vi "TDMS Write Through Publisher test.vi"() -> ()   [LabVIEW 2020]
uses:
  PPL/HDH.Actor Framework.Core.Publisher.lvlibp/Publisher/Publisher.lvclass
  C:/Current projects/WS/PPL/HDH.Actor Framework.Core.Actor.lvlibp/1abvi3w/vi.lib/ActorFramework/Actor/Actor.lvclass
  Actor/Dummy Actor/Dummy Actor.lvclass
  PPL/HDH.Actor Framework.Core.File Writer.lvlibp/File Writer Messages/Open File Msg/Open File Msg.lvclass
  C:/Current projects/WS/PPL/HDH.Actor Framework.Core.Actor.lvlibp/1abvi3w/vi.lib/ActorFramework/Message/Message.lvclass
  PPL/HDH.Actor Framework.Core.File Writer_TDMS.lvlibp/File Writer_TDMS/File Writer_TDMS.lvclass
  PPL/HDH.Data.Generic.lvlibp/Generic Data/Generic Array Data/Double Array/Double Array.lvclass
  C:/Current projects/WS/PPL/HDH.Data.Generic.lvlibp/Data.lvclass
  PPL/HDH.Actor Framework.Core.Publisher.lvlibp/Publisher Messages/Targetted Msg/Targetted Msg.lvclass
  PPL/HDH.Actor Framework.Core.Actor.lvlibp/1abvi3w/vi.lib/ActorFramework/Actor/Actor.lvclass
  PPL/HDH.Actor Framework.Core.Publisher.lvlibp/Publisher Messages/Launch Subscriber Msg/Launch Subscriber Msg.lvclass
  PPL/HDH.Actor Framework.Core.Actor.lvlibp
  PPL/HDH.Actor Framework.Core.Publisher.lvlibp/Publisher Messages/Publish Msg/Publish Msg.lvclass
  PPL/HDH.Actor Framework.Core.Actor.lvlibp/1abvi3w/vi.lib/ActorFramework/Stop Msg/Stop Msg.lvclass
  PPL/HDH.Actor Framework.Core.File Writer.lvlibp/File Writer/File Writer.lvclass
  PPL/HDH.Actor Framework.Core.Graph.lvlibp/Graph/Graph.lvclass
  C:/Current projects/WS/PPL/HDH.Actor Framework.Core.File Writer.lvlibp/File Writer/File Writer.lvclass
panel:
  in  "stop":bool
  out "error out":errorcluster
  in  "New File Path":path=path "C:/Current projects/HDH Framework/Test/TDMS Test Data.tdms"
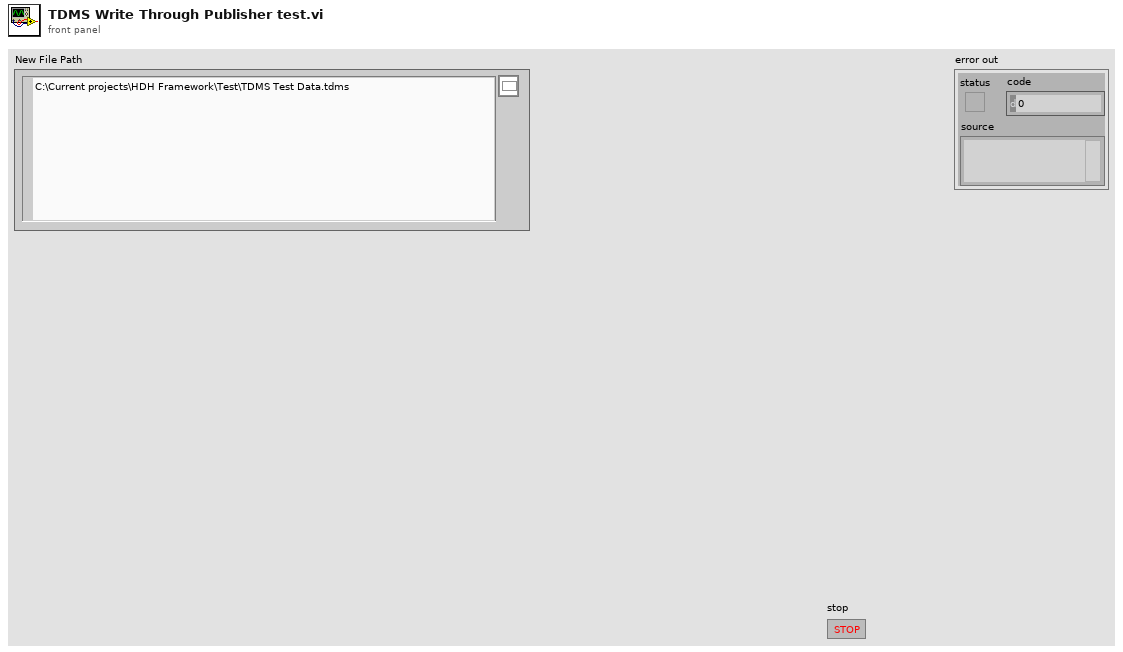
[diagram p1: front panel]
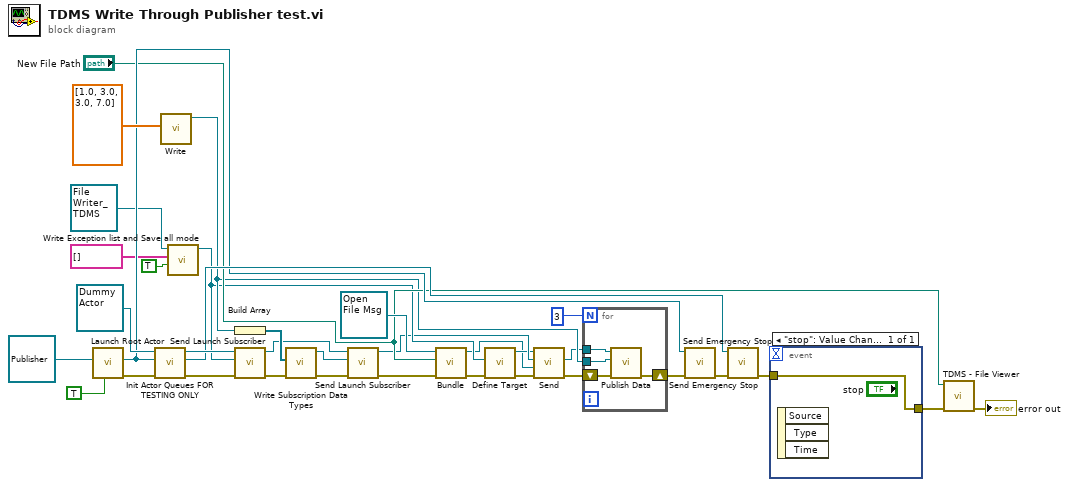
[diagram p0: block diagram]
diagram:
  n1 = call "Launch Root Actor.vi"("Open Actor Core front panel? (F)"=TRUE, "Actor"=refnum<class "Publisher.lvclass"> refnum ("HDH.Actor Framework.Core.Publisher.lvlibp:Publisher.lvclass")) -> ("error out"=w31:errorcluster, "Actor's Enqueuer"=w23:refnum<class "Message Enqueuer.lvclass">)  [unwired: 8 in]
  n2 = call "Init Actor Queues FOR TESTING ONLY.vi"("error in (no error)"=w31, "Actor-To-Caller Enqueuer"=w23, "Actor in"=refnum<class "Dummy Actor.lvclass"> refnum ("Test Actor.lvlib:Test Actor.lvclass")) -> ("error out"=w30:errorcluster, "Actor-To-Self Enqueuer"=w25:refnum<class "Message Enqueuer.lvclass">, "Actor out"=w33:refnum<class "Dummy Actor.lvclass">)  [unwired: 5 in, 1 out]
  n3 = call "Write.vi"("Double Array"=dbl[] [1.0, 3.0, 3.0, 7.0]) -> ("Double Array out"=w16:refnum<class "Double Array.lvclass">)  [unwired: 10 in]
  n4 = call "Write Exception list and Save all mode.vi"("Save all mode?"=TRUE, "Exception list"=string[] [], "File Writer in"=refnum<class "File Writer_TDMS.lvclass"> refnum ("HDH.Actor Framework.Core.File Writer_TDMS.lvlibp:File Writer_TDMS.lvclass")) -> ("File Writer out"=w9:refnum<class "File Writer_TDMS.lvclass">)  [unwired: 7 in, 1 out]
  n5 = Build Array(w16) -> (w15:refnum<class "Double Array.lvclass">[])
  n6 = call "Send Launch Subscriber.vi"("error in (no error)"=w30, "Actor to Launch"=w9, "Actor in"=w33) -> ("error out"=w12:errorcluster, "Actor out"=w14:refnum<class "Dummy Actor.lvclass">)  [unwired: 6 in, 1 out]
  n7 = call "Write Subscription Data Types.vi"("error in (no error)"=w12, "Subscription Data Types"=w15) -> ("error out"=w11:errorcluster, "Graph out"=w13:refnum<class "Graph.lvclass">)  [unwired: 8 in]
  n8 = call "Send Launch Subscriber.vi"("error in (no error)"=w11, "Actor to Launch"=w13, "Actor in"=w14) -> ("error out"=w10:errorcluster, "Actor out"=w7:refnum<class "Dummy Actor.lvclass">)  [unwired: 6 in, 1 out]
  n9 = call "Bundle.vi"("error in (no error)"=w10, "New File Path"="New File Path", "Open File Msg in"=refnum<class "Open File Msg.lvclass"> refnum) -> ("error out"=w8:errorcluster, "Open File Msg out"=w4:refnum<class "Open File Msg.lvclass">)  [unwired: 7 in]
  n10 = call "Define Target.vi"("error in (no error)"=w8, "Target Actor"=w9) -> ("error out"=w3:errorcluster, "Targetted Msg out"=w5:refnum<class "Targetted Msg.lvclass">)  [unwired: 8 in]
  n11 = call-dynamic "Send.vi"("error in (no error)"=w3, "Message"=w4, "Actor in"=w7, "Targetted Msg in"=w5) -> ("error out"=w2:errorcluster, "Actor out"=w6:refnum<class "Actor.lvclass">)  [unwired: 5 in, 1 out]
  n12 = for {
    N: 3 -> [_]
    tunnel: w6 -> [w39]
    tunnel: w16 -> [w38]
    shift-right: [w36] -> w27
    shift-left: w2 -> [w37]
    n13 = call "Publish Data.vi"("error in (no error)"=w37, "Data to Publish"=w38, "Actor in"=w39) -> ("error out"=w36:errorcluster)  [unwired: 6 in, 2 out]
  }
  n14 = call "Send Emergency Stop.vi"("error in (no error)"=w27, "Message Enqueuer"=w23) -> ("error out"=w26:errorcluster)  [unwired: 9 in]
  n15 = call "Send Emergency Stop.vi"("error in (no error)"=w26, "Message Enqueuer"=w25) -> ("error out"=w17:errorcluster)  [unwired: 9 in]
  n16 = event shown="[0] \"stop\": Value Change" {
    selector: _ -> [_]
    dyn-events: _ -> [_]
    timeout: _ -> [_]
    tunnel: [w40] -> w18
    tunnel: w17 -> [w40]
    event "stop": Value Change {
      n17 = event-data() -> ()  [unwired: 1 in, 3 out]
    }
  }
  n18 = call <vilib>:"TDMS - File Viewer.vi"("error in (no error)"=w18, "file path"="New File Path") -> ("error out"=→"error out":errorcluster)  [unwired: 4 in, 1 out]
